vi "PRACTICA 6.vi"() -> ()   [LabVIEW 2017]
panel:
  out "Numeric":i32
  out "x >= y?":bool
  in  "LIMITE":dbl
  in  "millisecond multiple":u32
  in  "stop":bool
  out "number (0 to 1)":dbl(slide) scale=0.0..100.0
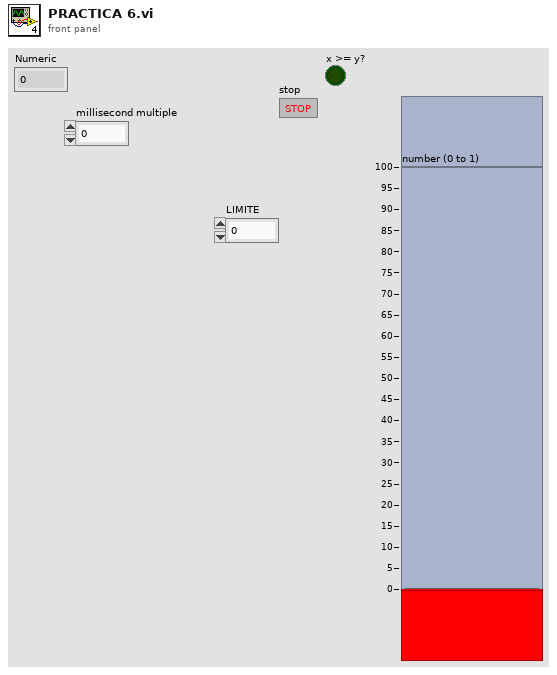
[diagram p1: front panel]
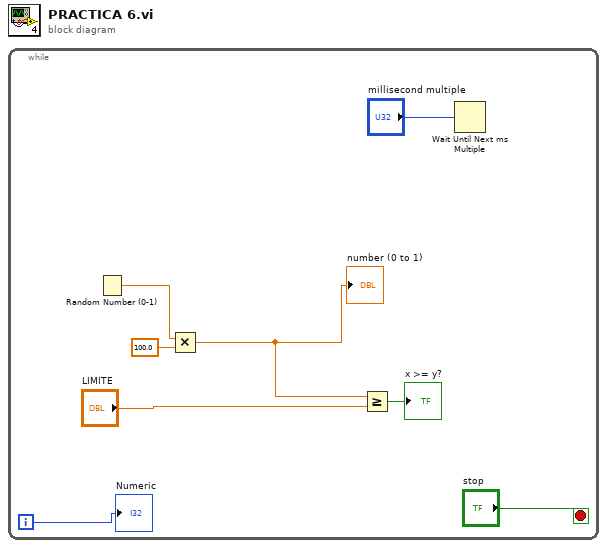
[diagram p0: block diagram]
diagram:
  n1 = while {
    i -> [w1]
    stop <- "stop" stop-if-true
    n2 = Random Number (0-1)() -> (number: 0 to 1=w6:dbl)
    n3 = Multiply(x=w6, y=100.0) -> (x*y=w4:dbl)
    "number (0 to 1)" <- w4
    n4 = Greater Or Equal?(x=w4, y="LIMITE") -> (x >= y?=→"x >= y?":bool)
    n5 = Wait Until Next ms Multiple(millisecond multiple="millisecond multiple") -> ()  [unwired: 1 out]
    "Numeric" <- w1
  }
